vi "LoadData.vi"(1 "Data File":path=path "G:/Data") -> (0 "Data":string[][](table))   [LabVIEW 2014]
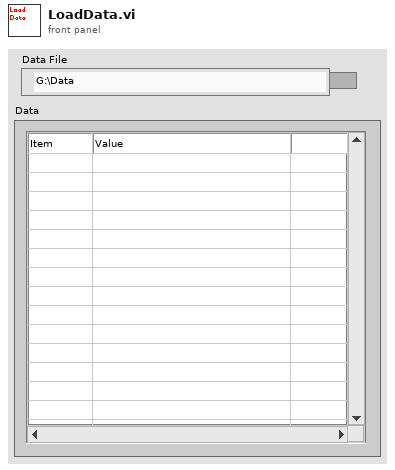
[diagram p1: front panel]
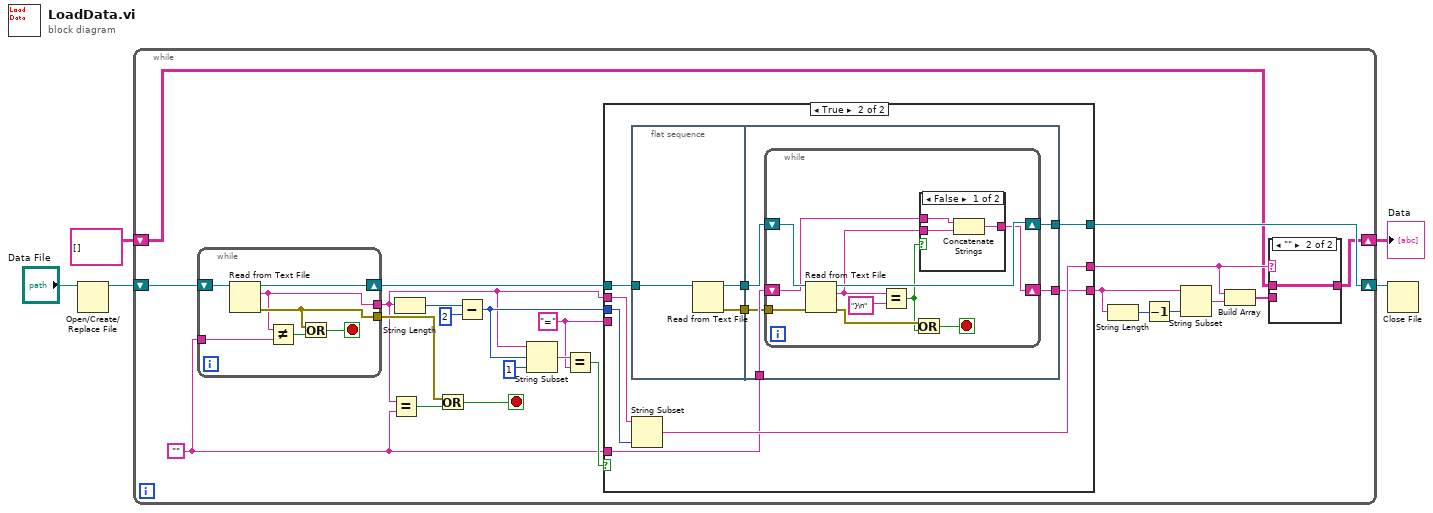
[diagram p0: block diagram]
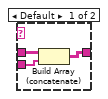
[diagram p2: hidden frame]
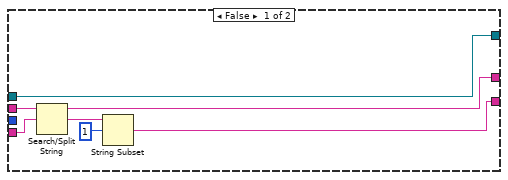
[diagram p3: hidden frame]
diagram:
  n1 = Open/Create/Replace File(file path (use dialog)="Data File") -> (refnum out=w5:refnum<file>)  [unwired: 5 in, 2 out]
  n2 = while {
    shift-right: [w21] -> w1
    shift-left: w5 -> [w15]
    shift-right: [w6] -> w3
    shift-left: string[][] [] -> [w7]
    stop <- w11 stop-if-true
    w10 = ""
    w22 = "=" ("y")
    n3 = while {
      tunnel: [w37] -> w13
      shift-right: [w39] -> w16
      shift-left: w15 -> [w35]
      tunnel: [w38] -> w14
      tunnel: w10 -> [w33]
      stop <- w34 stop-if-true
      n4 = Read from Text File(file (use dialog)=w35) -> (refnum out=w39:refnum<file>, text=w37:string, error out=w38:errorcluster)  [unwired: 3 in, 1 out]
      n5 = Not Equal?(x=w37, y=w33) -> (x != y?=w36:bool)
      n6 = Or(x=w38, y=w36) -> (x .or. y?=w34:bool)
    }
    n7 = Equal?(x=w13, y=w10) -> (x = y?=w12:bool)
    n8 = String Length(string=w13) -> (length=w26:i32)
    n9 = Or(x=w14, y=w12) -> (x .or. y?=w11:bool)
    n10 = Subtract(x=w26, y=2) -> (x-y=w27:i32)
    n11 = String Subset(string=w13, offset (0)=w27, length (rest)=1 ("length (rest)")) -> (substring=w24:string)
    n12 = Equal?(x=w24, y=w22) -> (x = y?=w28:bool)
    n13 = case shown="True" w28 {
      tunnel: w13 -> [w46 w55]
      tunnel: w27 -> [_ w54]
      tunnel: [w44 w53] -> w9
      tunnel: w22 -> [w45 _]
      tunnel: [w40 w49] -> w18
      tunnel: w16 -> [w43 w52]
      tunnel: [w43 w51] -> w21
      tunnel: w10 -> [_ w48]
      frame False {
        n14 = Search/Split String(string=w46, search string/char (-)=w45) -> (substring before match=w44:string, match + rest of string=w42:string)  [unwired: 1 in, 1 out]
        n15 = String Subset(string=w42, offset (0)=1) -> (substring=w40:string)  [unwired: 1 in]
      }
      frame True {
        n16 = flat-sequence {
          tunnel: w52 -> [w58]
          tunnel: [w57] -> w50
          tunnel: [w56] -> w47
          tunnel: [w62] -> w51
          tunnel: w50 -> [w63]
          tunnel: [w61] -> w49
          tunnel: w48 -> [w60]
          tunnel: w47 -> [w59]
          frame #0 {
            n17 = Read from Text File(file (use dialog)=w58) -> (refnum out=w57:refnum<file>, error out=w56:errorcluster)  [unwired: 3 in, 2 out]
          }
          frame #1 {
            n18 = while {
              shift-right: [w72] -> w62
              shift-left: w63 -> [w73]
              shift-right: [w69] -> w61
              shift-left: w60 -> [w68]
              tunnel: w59 -> [w67]
              stop <- w66 stop-if-true
              n19 = Read from Text File(file (use dialog)=w73, error in=w67) -> (refnum out=w72:refnum<file>, text=w70:string, error out=w65:errorcluster)  [unwired: 2 in, 1 out]
              n20 = Equal?(x=w70, y="}\n") -> (x = y?=w64:bool)
              n21 = Or(x=w65, y=w64) -> (x .or. y?=w66:bool)
              n22 = case shown="False" w64 {
                tunnel: [w74 w77] -> w69
                tunnel: w70 -> [w75 _]
                tunnel: w68 -> [w76 w77]
                frame False {
                  n23 = Concatenate Strings(w76, w75) -> (w74:string)
                }
                frame True {
                }
              }
            }
          }
        }
        n24 = String Subset(string=w55, length (rest)=w54) -> (substring=w53:string)  [unwired: 1 in]
      }
    }
    n25 = String Length(string=w18) -> (length=w20:i32)
    n26 = Decrement(x=w20) -> (x-1=w19:i32)
    n27 = String Subset(string=w18, length (rest)=w19) -> (substring=w17:string)  [unwired: 1 in]
    n28 = Build Array(w9, w17) -> (w8:string[])
    n29 = case shown="\"\"" w9 {
      tunnel: w8 -> [w31 _]
      tunnel: w7 -> [w30 w32]
      tunnel: [w29 w32] -> w6
      frame Default {
        n30 = Build Array (concatenate)(w30, w31) -> (w29:string[][])
      }
      frame "" {
      }
    }
  }
  "Data" <- w3
  n31 = Close File(refnum=w1) -> ()  [unwired: 1 in, 2 out]
